vi "IoT_RESTful.vi"(6 "Method":enum16{"GET", "PUT", "POST", "MultiPOST"}(ring), 7 "url":string, 8 "error in":errorcluster, 9 "data":T1[](array[typedef]), 10 "JSON":string, 11 "Device In":T3={"Name"="", "BaseURL"="", "AppKey"="", "Headers"=["Content-Type:application/json"], "Timeout"=10000, "Identifier"="", "Password"="", "Comments"="", "Handle"=0, "# Handles"=0}) -> (0 "error out":errorcluster, 1 "HTTP Code":i32, 2 "Comm":T2, 3 "Device Out":T3={"Name"="", "BaseURL"="", "AppKey"="", "Headers"=["Content-Type:application/json"], "Timeout"=10000, "Identifier"="", "Password"="", "Comments"="", "Handle"=0, "# Handles"=0})   [LabVIEW 2016]
uses:
  <vilib>/httpClient/LabVIEWHTTPClient.lvlib
  <vilib>/httpClient/PUTBuffer.vi
  RWPrefCluster.vi
  <vilib>/httpClient/POSTBuffer.vi
  Device.ctl
  HTTPComm.ctl
  <vilib>/httpClient/MultipartData.ctl
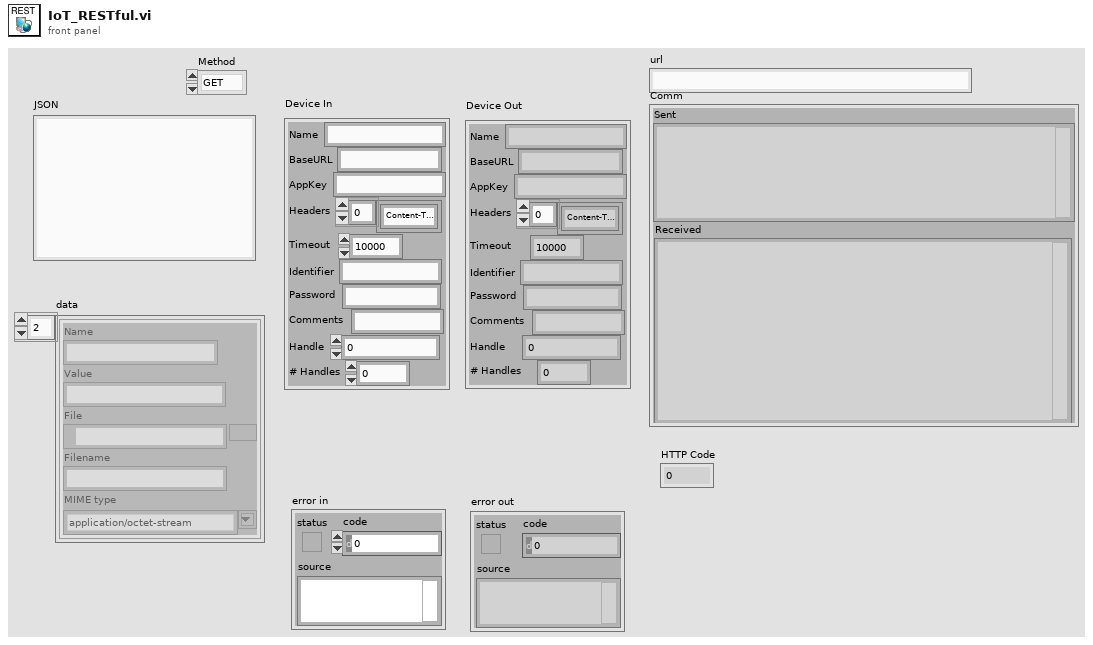
[diagram p1: front panel]
types:
  T1 = typedef "LabVIEWHTTPClient.lvlib/MultipartData.ctl" = cluster{"Name":string, "Value":string, "File":path, "Filename":string, "MIME type":string}
  T2 = typedef "HTTPComm.ctl" = cluster{"url":string, "sent headers":string, "sent body":string, "headers":string, "body":string, "Sent":string, "Received":string}
  T3 = typedef "Device.ctl" = cluster{"Name":string, "BaseURL":string, "AppKey":string, "Headers":string[], "Timeout":i32, "Identifier":string, "Password":string, "Comments":string, "Handle":u32, "# Handles":i32}
  T4 = typedef "LabVIEWHTTPClient.lvlib/ClientHandle.ctl" = refnum<k1>
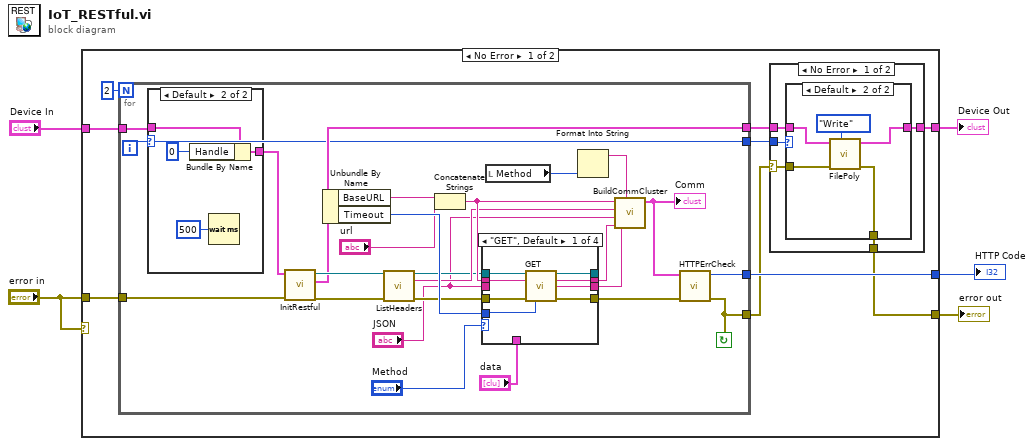
[diagram p0: block diagram]
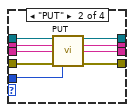
[diagram p5: hidden frame]
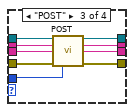
[diagram p6: hidden frame]
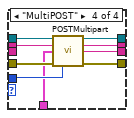
[diagram p7: hidden frame]
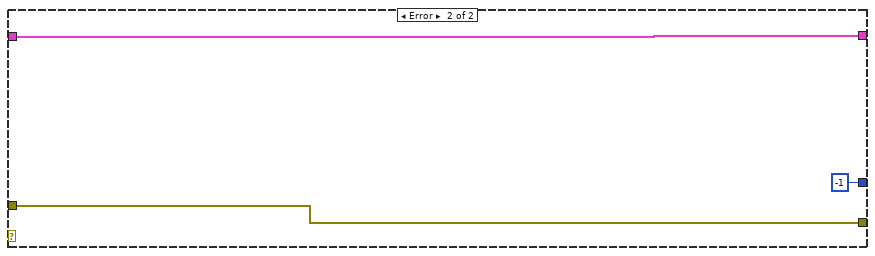
[diagram p8: hidden frame]
diagram:
  n1 = case shown="No Error" "error in" {
    tunnel: "error in" -> [w12 w95]
    tunnel: "Device In" -> [w11 w96]
    tunnel: [w8 w96] -> w4
    tunnel: [w6 w95] -> w3
    tunnel: [w14 -1 ("error")] -> w1
    frame No Error {
      n2 = for {
        N: 2 -> [_]
        tunnel: [w35] -> w14
        tunnel: w12 -> [w32]
        tunnel: [w34] -> w7
        tunnel: [w33] -> w9
        tunnel: w11 -> [w30]
        tunnel: [w29] -> w10
        i -> [w29]
        stop <- w34 continue-if-true
        n3 = case shown="Default" w29 {
          tunnel: w30 -> [w54 w57]
          tunnel: [w54 w56] -> w31
          frame 0 {
          }
          frame Default {
            n4 = Bundle By Name(cluster=w57, "Handle"=u32 0) -> (w56:T3)
            n5 = Wait (ms)(milliseconds to wait=u32 500) -> ()  [unwired: 1 out]
          }
        }
        n6 = call "InitRestful.vi"("error in (no error)"=w32, "Device In"=w31) -> ("error out"=w46:errorcluster, "Device Out"=w33:T3, "Refnum out"=w47:T4)  [unwired: 7 in]
        n7 = Unbundle By Name(w33) -> ("BaseURL"=w43:string, "Timeout"=w52:i32)
        n8 = call <vilib>:"ListHeaders.vi"("client handle"=w47, "error in (no error)"=w46) -> ("client handle out"=w48:T4, "headers"=w50:string, "error out"=w49:errorcluster)  [unwired: 11 in]
        n9 = Concatenate Strings(w43, "url") -> (w51:string)
        n10 = case shown="\"GET\", Default" "Method" {
          tunnel: [w66 w75 w84 w93] -> w53
          tunnel: [w65 w74 w83 w92] -> w37
          tunnel: [w64 w73 w82 w91] -> w38
          tunnel: w52 -> [w63 w72 w81 w90]
          tunnel: w51 -> [w62 w71 w80 w89]
          tunnel: w49 -> [w61 w70 w79 w88]
          tunnel: w48 -> [w60 w69 w78 w87]
          tunnel: "JSON" -> [_ w68 w77 _]
          tunnel: [w59 w67 w76 w86] -> _
          tunnel: "data" -> [_ _ _ w85]
          frame "GET", Default {
            n11 = call <vilib>:"GET.vi"("client handle"=w60, "url"=w62, "error in (no error)"=w61, "timeout (10000)"=w63) -> ("client handle out"=w59:T4, "headers"=w66:string, "body"=w65:string, "error out"=w64:errorcluster)  [unwired: 8 in]
          }
          frame "PUT" {
            n12 = call-poly <vilib>:"PUT.vi"("client handle"=w69, "url"=w71, "buffer"=w68, "error in (no error)"=w70, "timeout (10000)"=w72) -> ("client handle out"=w67:T4, "headers"=w75:string, "body"=w74:string, "error out"=w73:errorcluster)  [unwired: 7 in]
          }
          frame "POST" {
            n13 = call-poly <vilib>:"POST.vi"("client handle"=w78, "url"=w80, "buffer"=w77, "error in (no error)"=w79, "timeout (10000)"=w81) -> ("client handle out"=w76:T4, "headers"=w84:string, "body"=w83:string, "error out"=w82:errorcluster)  [unwired: 7 in]
          }
          frame "MultiPOST" {
            n14 = call <vilib>:"POSTMultipart.vi"("client handle"=w87, "url"=w89, "data"=w85, "error in (no error)"=w88, "timeout (10000)"=w90) -> ("client handle out"=w86:T4, "headers"=w93:string, "body"=w92:string, "error out"=w91:errorcluster)  [unwired: 7 in]
          }
        }
        n15 = local read "Method"() -> (w41:enum16{"GET", "PUT", "POST", "MultiPOST"})
        n16 = Format Into String(w41) -> (resulting string=w40:string)  [unwired: 3 in, 1 out]
        n17 = call "BuildCommCluster.vi"("reply body"=w37, "Type"=w40, "reply headers"=w53, "sent body"="JSON", "sent headers"=w50, "url"=w51) -> ("Comm"=w36:T2)  [unwired: 5 in]
        "Comm" <- w36
        n18 = call "HTTPErrCheck.vi"("error in (no error)"=w38, "Comm"=w36) -> ("error out"=w34:errorcluster, "error"=w35:i32)  [unwired: 8 in]
      }
      n19 = case shown="No Error" w7 {
        selector: w7 -> [w15 w27]
        tunnel: w10 -> [w19 _]
        tunnel: w9 -> [w18 w28]
        tunnel: [w17 w28] -> w8
        tunnel: [w16 w27] -> w6
        frame No Error {
          n20 = case shown="Default" w19 {
            tunnel: w18 -> [w21 w26]
            tunnel: [w21 w25] -> w17
            tunnel: [w20 w23] -> w16
            tunnel: w15 -> [w20 w22]
            frame 0 {
            }
            frame Default {
              n21 = call-poly "FilePoly.vi"("Task"=enum16{"Read", "Write"}."Write", "error in (no error)"=w22, "Device In"=w26) -> ("error out"=w23:errorcluster, "Device Out"=w25:T3)  [unwired: 7 in]
            }
          }
        }
        frame Error {
        }
      }
    }
    frame Error {
    }
  }
  "error out" <- w3
  "Device Out" <- w4
  "HTTP Code" <- w1
